vi "6300 laser sweep example.vi"() -> ()   [LabVIEW 2011]
panel:
  out "error out":errorcluster
  out "WavelengthMin":dbl format="%.2f"
  out "WavelengthMax":dbl format="%.2f"
  out "MaxSlewRate":dbl format="%.2f"
  in  "StartSweep":bool
  in  "ReturnSlewrate":dbl format="%.2f"
  in  "ForwardSlewrate":dbl format="%.2f"
  in  "StopWavelength":dbl format="%.2f"
  in  "StartWavelength":dbl format="%.2f"
  in  "resource name (\"\")":string="GPIB0::10::INSTR"
  # "Sweep Example\n\nStart program with above arrow.\nSet parameters and press StartSweep.\nLaser will reset to the start wavelength then sweep to the stop wavelength."
  # "Min"
  # "Max"
  # "Max"
  # "Set up for GPIB address 1.  Change as needed."
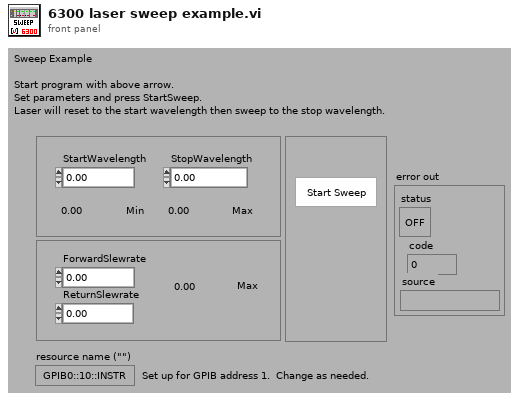
[diagram p1: front panel]
types:
  T1 = enum16{"Diode Current", "Diode Temperature", "Piezo Volt", "Wavelength", "Forward Slew Rate", "Return Slew Rate", "Scan Start Wavelength", "Scan Stop Wavelength", "MaxSlewRate", "Wavelength Max", "Wavelength Min"}
  T2 = enum16{"Diode Current", "Diode Temperature", "Piezo Volt", "Wavelength", "Forward Slewrate", "Return Slewrate", "Scan Start Wavelength", "Scan Stop Wavelength", "Wavelength Max", "Wavelength Min", "Constant Power On", "Constant Power Off"}
  T3 = enum16{"Scan Reset", "Scan Start", "Scan Stop", "Laser On", "Laser Off", "Laser State?", "Track Off"}
  T4 = enum16{"Identification Query", "Operation Complete Query"}
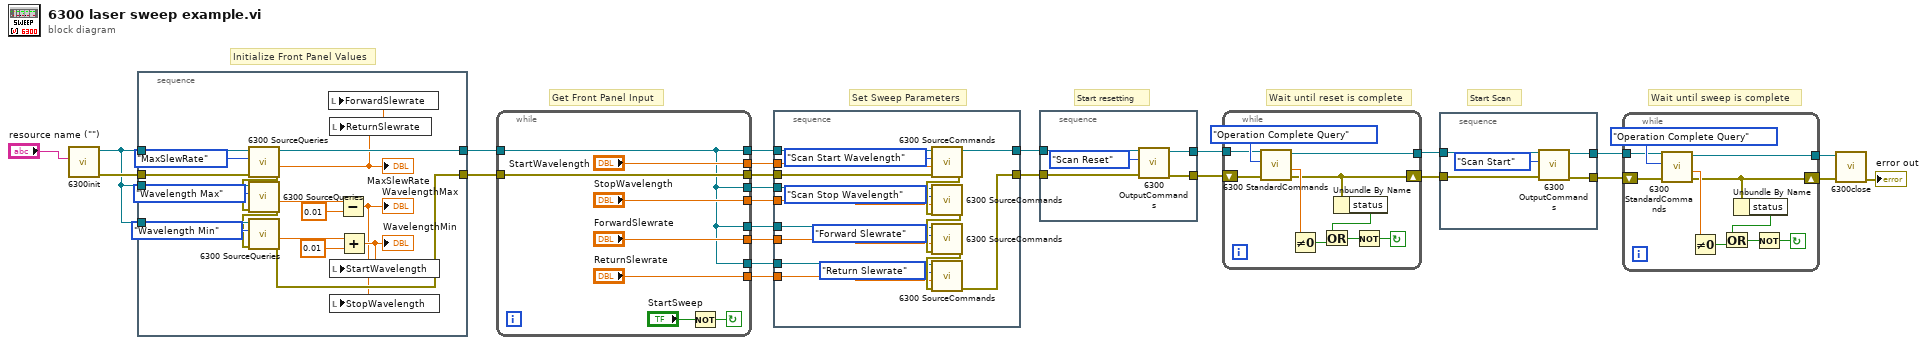
[diagram p0: block diagram]
diagram:
  # "Initialize Front Panel Values"
  # "Wait until sweep is complete"
  # "Start Scan"
  # "Wait until reset is complete"
  # "Start resetting"
  # "Set Sweep Parameters"
  # "Get Front Panel Input"
  n1 = call <instrlib>:"6300init.vi"("resource name (\"\")"="resource name (\"\")") -> ("error out"=w5:errorcluster, "dup VISA session"=w2:refnum<visa-resource-name>)  [unwired: 9 in]
  n2 = stacked-sequence {
    tunnel: w2 -> [w39]
    tunnel: w5 -> [w38]
    tunnel: [w39] -> w4
    tunnel: [w33] -> w3
    tunnel: w2 -> [w37]
    tunnel: w2 -> [w36]
    frame #0 {
      n3 = call <instrlib>:"6300 SourceQueries.VI"("error in"=w38, "Setpoint to Query?"=T1."MaxSlewRate", "VISA session"=w39) -> ("error out"=w35:errorcluster, "Returned Number"=w26:dbl)  [unwired: 5 in, 2 out]
      "MaxSlewRate" <- w26
      n4 = call <instrlib>:"6300 SourceQueries.VI"("error in"=w35, "Setpoint to Query?"=T1."Wavelength Max", "VISA session"=w37) -> ("error out"=w34:errorcluster, "Returned Number"=w29:dbl)  [unwired: 5 in, 2 out]
      n5 = call <instrlib>:"6300 SourceQueries.VI"("error in"=w34, "Setpoint to Query?"=T1."Wavelength Min", "VISA session"=w36) -> ("error out"=w33:errorcluster, "Returned Number"=w30:dbl)  [unwired: 5 in, 2 out]
      n6 = local write "ForwardSlewrate"(w26) -> ()
      n7 = local write "ReturnSlewrate"(w26) -> ()
      n8 = Subtract(x=w29, y=0.01) -> (x-y=w27:dbl)
      "WavelengthMax" <- w27
      n9 = local write "StopWavelength"(w27) -> ()
      n10 = Add(x=w30, y=0.01) -> (x+y=w28:dbl)
      "WavelengthMin" <- w28
      n11 = local write "StartWavelength"(w28) -> ()
    }
  }
  n12 = while {
    tunnel: [w43] -> w16
    tunnel: [w43] -> w17
    tunnel: [w43] -> w18
    tunnel: [w43] -> w19
    tunnel: ["ReturnSlewrate"] -> w21
    tunnel: ["ForwardSlewrate"] -> w22
    tunnel: ["StopWavelength"] -> w23
    tunnel: ["StartWavelength"] -> w24
    tunnel: [w50] -> w20
    tunnel: w3 -> [w50]
    tunnel: w4 -> [w43]
    stop <- w44 continue-if-true
    n13 = Not(x="StartSweep") -> (.not. x?=w44:bool)
  }
  n14 = stacked-sequence {
    tunnel: w24 -> [w65]
    tunnel: w23 -> [w64]
    tunnel: w22 -> [w63]
    tunnel: w21 -> [w62]
    tunnel: w20 -> [w61]
    tunnel: [w60] -> w14
    tunnel: w19 -> [w59]
    tunnel: w18 -> [w58]
    tunnel: w17 -> [w57]
    tunnel: w16 -> [w56]
    tunnel: [w55] -> w15
    frame #0 {
      n15 = call <instrlib>:"6300 SourceCommands.VI"("error in"=w61, "Num Com Parameter"=w65, "Source Command?"=T2."Scan Start Wavelength", "VISA session"=w59) -> ("error out"=w68:errorcluster, "dup VISA session"=w55:refnum<visa-resource-name>)  [unwired: 4 in, 2 out]
      n16 = call <instrlib>:"6300 SourceCommands.VI"("error in"=w68, "Num Com Parameter"=w64, "Source Command?"=T2."Scan Stop Wavelength", "VISA session"=w58) -> ("error out"=w67:errorcluster)  [unwired: 4 in, 3 out]
      n17 = call <instrlib>:"6300 SourceCommands.VI"("error in"=w67, "Num Com Parameter"=w63, "Source Command?"=T2."Forward Slewrate", "VISA session"=w57) -> ("error out"=w66:errorcluster)  [unwired: 4 in, 3 out]
      n18 = call <instrlib>:"6300 SourceCommands.VI"("error in"=w66, "Num Com Parameter"=w62, "Source Command?"=T2."Return Slewrate", "VISA session"=w56) -> ("error out"=w60:errorcluster)  [unwired: 4 in, 3 out]
    }
  }
  n19 = stacked-sequence {
    tunnel: w15 -> [w73]
    tunnel: w14 -> [w72]
    tunnel: [w70] -> w13
    tunnel: [w69] -> w12
    frame #0 {
      n20 = call <instrlib>:"6300 OutputCommands.VI"("error in"=w72, "Output Command?"=T3."Scan Reset", "VISA session"=w73) -> ("error out"=w70:errorcluster, "dup VISA session"=w69:refnum<visa-resource-name>)  [unwired: 3 in, 4 out]
    }
  }
  n21 = while {
    tunnel: [w76] -> w9
    tunnel: w12 -> [w80]
    shift-left: w13 -> [w79]
    shift-right: [w75] -> w8
    stop <- w78 continue-if-true
    n22 = call <instrlib>:"6300 StandardCommands.VI"("error in"=w79, "System Command?"=T4."Operation Complete Query", "VISA session"=w80) -> ("error out"=w75:errorcluster, "Returned Number"=w81:dbl, "dup VISA session"=w76:refnum<visa-resource-name>)  [unwired: 5 in, 1 out]
    n23 = Not Equal To 0?(x=w81) -> (x != 0?=w82:bool)
    n24 = Unbundle By Name(w75) -> ("status"=w74:bool)
    n25 = Or(x=w74, y=w82) -> (x .or. y?=w77:bool)
    n26 = Not(x=w77) -> (.not. x?=w78:bool)
  }
  n27 = stacked-sequence {
    tunnel: w9 -> [w88]
    tunnel: w8 -> [w87]
    tunnel: [w85] -> w10
    tunnel: [w84] -> w11
    frame #0 {
      n28 = call <instrlib>:"6300 OutputCommands.VI"("error in"=w87, "Output Command?"=T3."Scan Start", "VISA session"=w88) -> ("error out"=w85:errorcluster, "dup VISA session"=w84:refnum<visa-resource-name>)  [unwired: 3 in, 4 out]
    }
  }
  n29 = while {
    tunnel: [w91] -> w7
    tunnel: w11 -> [w95]
    shift-left: w10 -> [w94]
    shift-right: [w90] -> w6
    stop <- w93 continue-if-true
    n30 = call <instrlib>:"6300 StandardCommands.VI"("error in"=w94, "System Command?"=T4."Operation Complete Query", "VISA session"=w95) -> ("error out"=w90:errorcluster, "Returned Number"=w96:dbl, "dup VISA session"=w91:refnum<visa-resource-name>)  [unwired: 5 in, 1 out]
    n31 = Not Equal To 0?(x=w96) -> (x != 0?=w97:bool)
    n32 = Unbundle By Name(w90) -> ("status"=w89:bool)
    n33 = Or(x=w89, y=w97) -> (x .or. y?=w92:bool)
    n34 = Not(x=w92) -> (.not. x?=w93:bool)
  }
  n35 = call <instrlib>:"6300close.vi"("error in"=w6, "VISA session"=w7) -> ("error out"=→"error out":errorcluster)  [unwired: 9 in]
